vi "Edit-dialog.vi"(8 "error in (no error)":errorcluster, 11 "Action in":refnum<class "Action.lvclass">) -> (0 "error out":errorcluster, 3 "Action out":refnum<class "Action.lvclass">)   [LabVIEW 2013, in "PowderDeposition.lvlib" / "Action.lvclass"]
uses:
  Action.lvclass
panel:
  in  "Cancel":bool
  in  "OK":bool
  in  "Edit dialog":cluster{"Nothing editable":string}
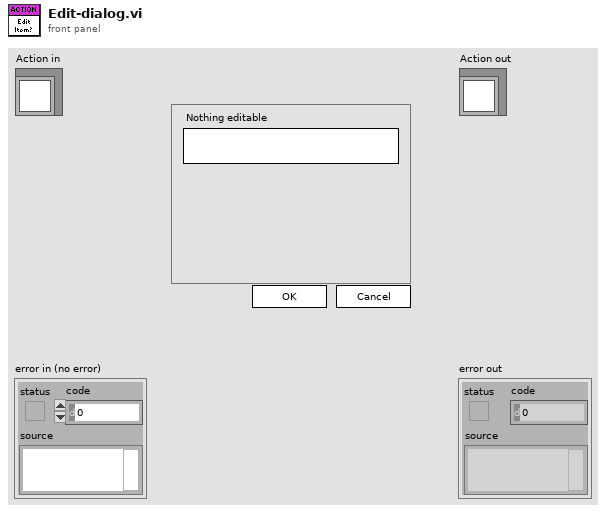
[diagram p1: front panel]
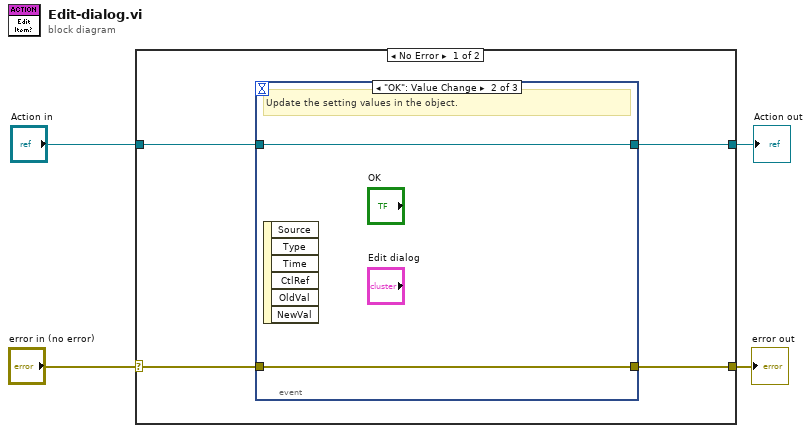
[diagram p0: block diagram]
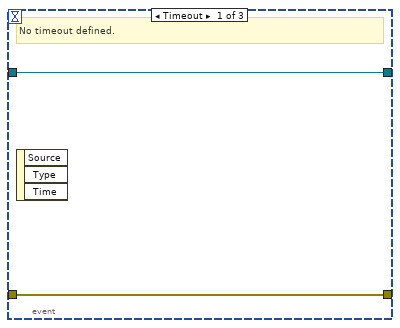
[diagram p2: hidden frame]
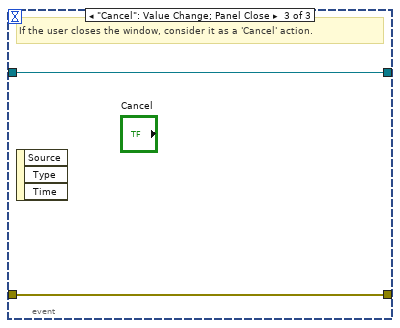
[diagram p3: hidden frame]
diagram:
  n1 = case shown="No Error" "error in (no error)" {
    selector: "error in (no error)" -> [w6 w16]
    tunnel: [w5 w16] -> w3
    tunnel: [w7 w15] -> w1
    tunnel: "Action in" -> [w8 w15]
    frame No Error {
      n2 = event shown="[1] \"OK\": Value Change" {
        selector: _ -> [_ _ _]
        dyn-events: _ -> [_ _ _]
        timeout: _ -> [_ _ _]
        tunnel: w8 -> [w10 w12 w14]
        tunnel: [w10 w12 w14] -> w7
        tunnel: w6 -> [w9 w11 w13]
        tunnel: [w9 w11 w13] -> w5
        event Timeout {
          # "No timeout defined."
          n3 = event-data() -> ()  [unwired: 1 in, 3 out]
        }
        event "OK": Value Change {
          # "Update the setting values in the object."
          n4 = event-data() -> ()  [unwired: 1 in, 6 out]
        }
        event "Cancel": Value Change; Panel Close {
          # "If the user closes the window, consider it as a 'Cancel' action."
          n5 = event-data() -> ()  [unwired: 1 in, 3 out]
        }
      }
    }
    frame Error {
    }
  }
  "error out" <- w3
  "Action out" <- w1
